vi "Global Controls.vi"() -> ()   [LabVIEW 2020]
uses:
  _controls/PCIe SLM params.ctl
  _controls/PCIe SLM Spots.ctl
  _controls/Spot Params.ctl
  _controls/Exp Params.ctl
  _controls/Global Ctrl Refs.ctl
  _controls/Trapping Laser Control.ctl
  _controls/xiCam.ctl
  <vilib>/userDefined/High Color/IMAQdx.ctl
  _controls/SLM Real World to IMAQ Display Transform.ctl
panel:
  in  "SLM to IMAQ":T1={"Translation"={"X"=255.9856, "Y"=245.976}, "Scalling"={"xScale"=2.61758691206544, "yScale"=-2.61759}}
  in  "Camera Controls":T2={"Exposure Time (ms)"=27, "cam0 Session"="", "Camera ROI"={"Width"=0, "Height"=0, "Offset X"=0, "Offset Y"=0}, "Command"=""} {"Camera ROI"."Offset Y" max=2046 step=2; "Camera ROI"."Offset X" max=2044 step=4; "Camera ROI"."Height" min=2 max=2048 step=2; "Camera ROI"."Width" min=4 max=2048 step=4; "Exposure Time (ms)" min=27 max=500 step=1 scale=27.0..500.0}
  in  "Ventus Controls":T4 caption="Trapping Laser" {"Ventus Power" min=0.0 max=100.0 step=0.1 scale=0.0..100.0}
  in  "Global Ctrl Refs":T5
  in  "Exp Params":T6={"Experiment Type"="Time Series", "Experiment Name"="Experiment_1", "ExpPath"=path "D:/Data", "Save As"="Time Series", "TSFrames"=1000, "TSfps"=1000.0, "Streaming"=FALSE, "tdms ref"=refnum, "frame #"=0, "Full Path"=path "", "PeakOnQueue"=FALSE} {"TSFrames" min=1 step=1; "TSfps" min=0.001 max=90.0 step=0.001 format="%_4g"}
  out "holo_combine":u8[](array[numeric])
  in  "Spots":T7={"Spot Params"=[{"Intensity"=1.0, "Vortex"=0.0, "Phase"=0.0, "X"=0.0, "Y"=0.0, "Z"=0.0}], "Add Spot"=FALSE, "Remove Spot"=FALSE, "Clear All Spots"=FALSE, "Save Spots"=FALSE, "Generate Spots"=FALSE, "Generate Spot Pattern"=""} {"Spot Params"."Z" format="%_4g"; "Spot Params"."Y" format="%_4g"; "Spot Params"."X" format="%_4g"; "Spot Params"."Phase" format="%_4g"; "Spot Params"."Intensity" format="%_4g"}
  out "SLM Params":T9={"Width"=0.0, "Height"=0.0, "Board ID"=0, "Centre Y"=0.46199999999999997, "Centre X"=0.3859999999999999} {"Centre X" format="%.3g"; "Centre Y" format="%.3g"}
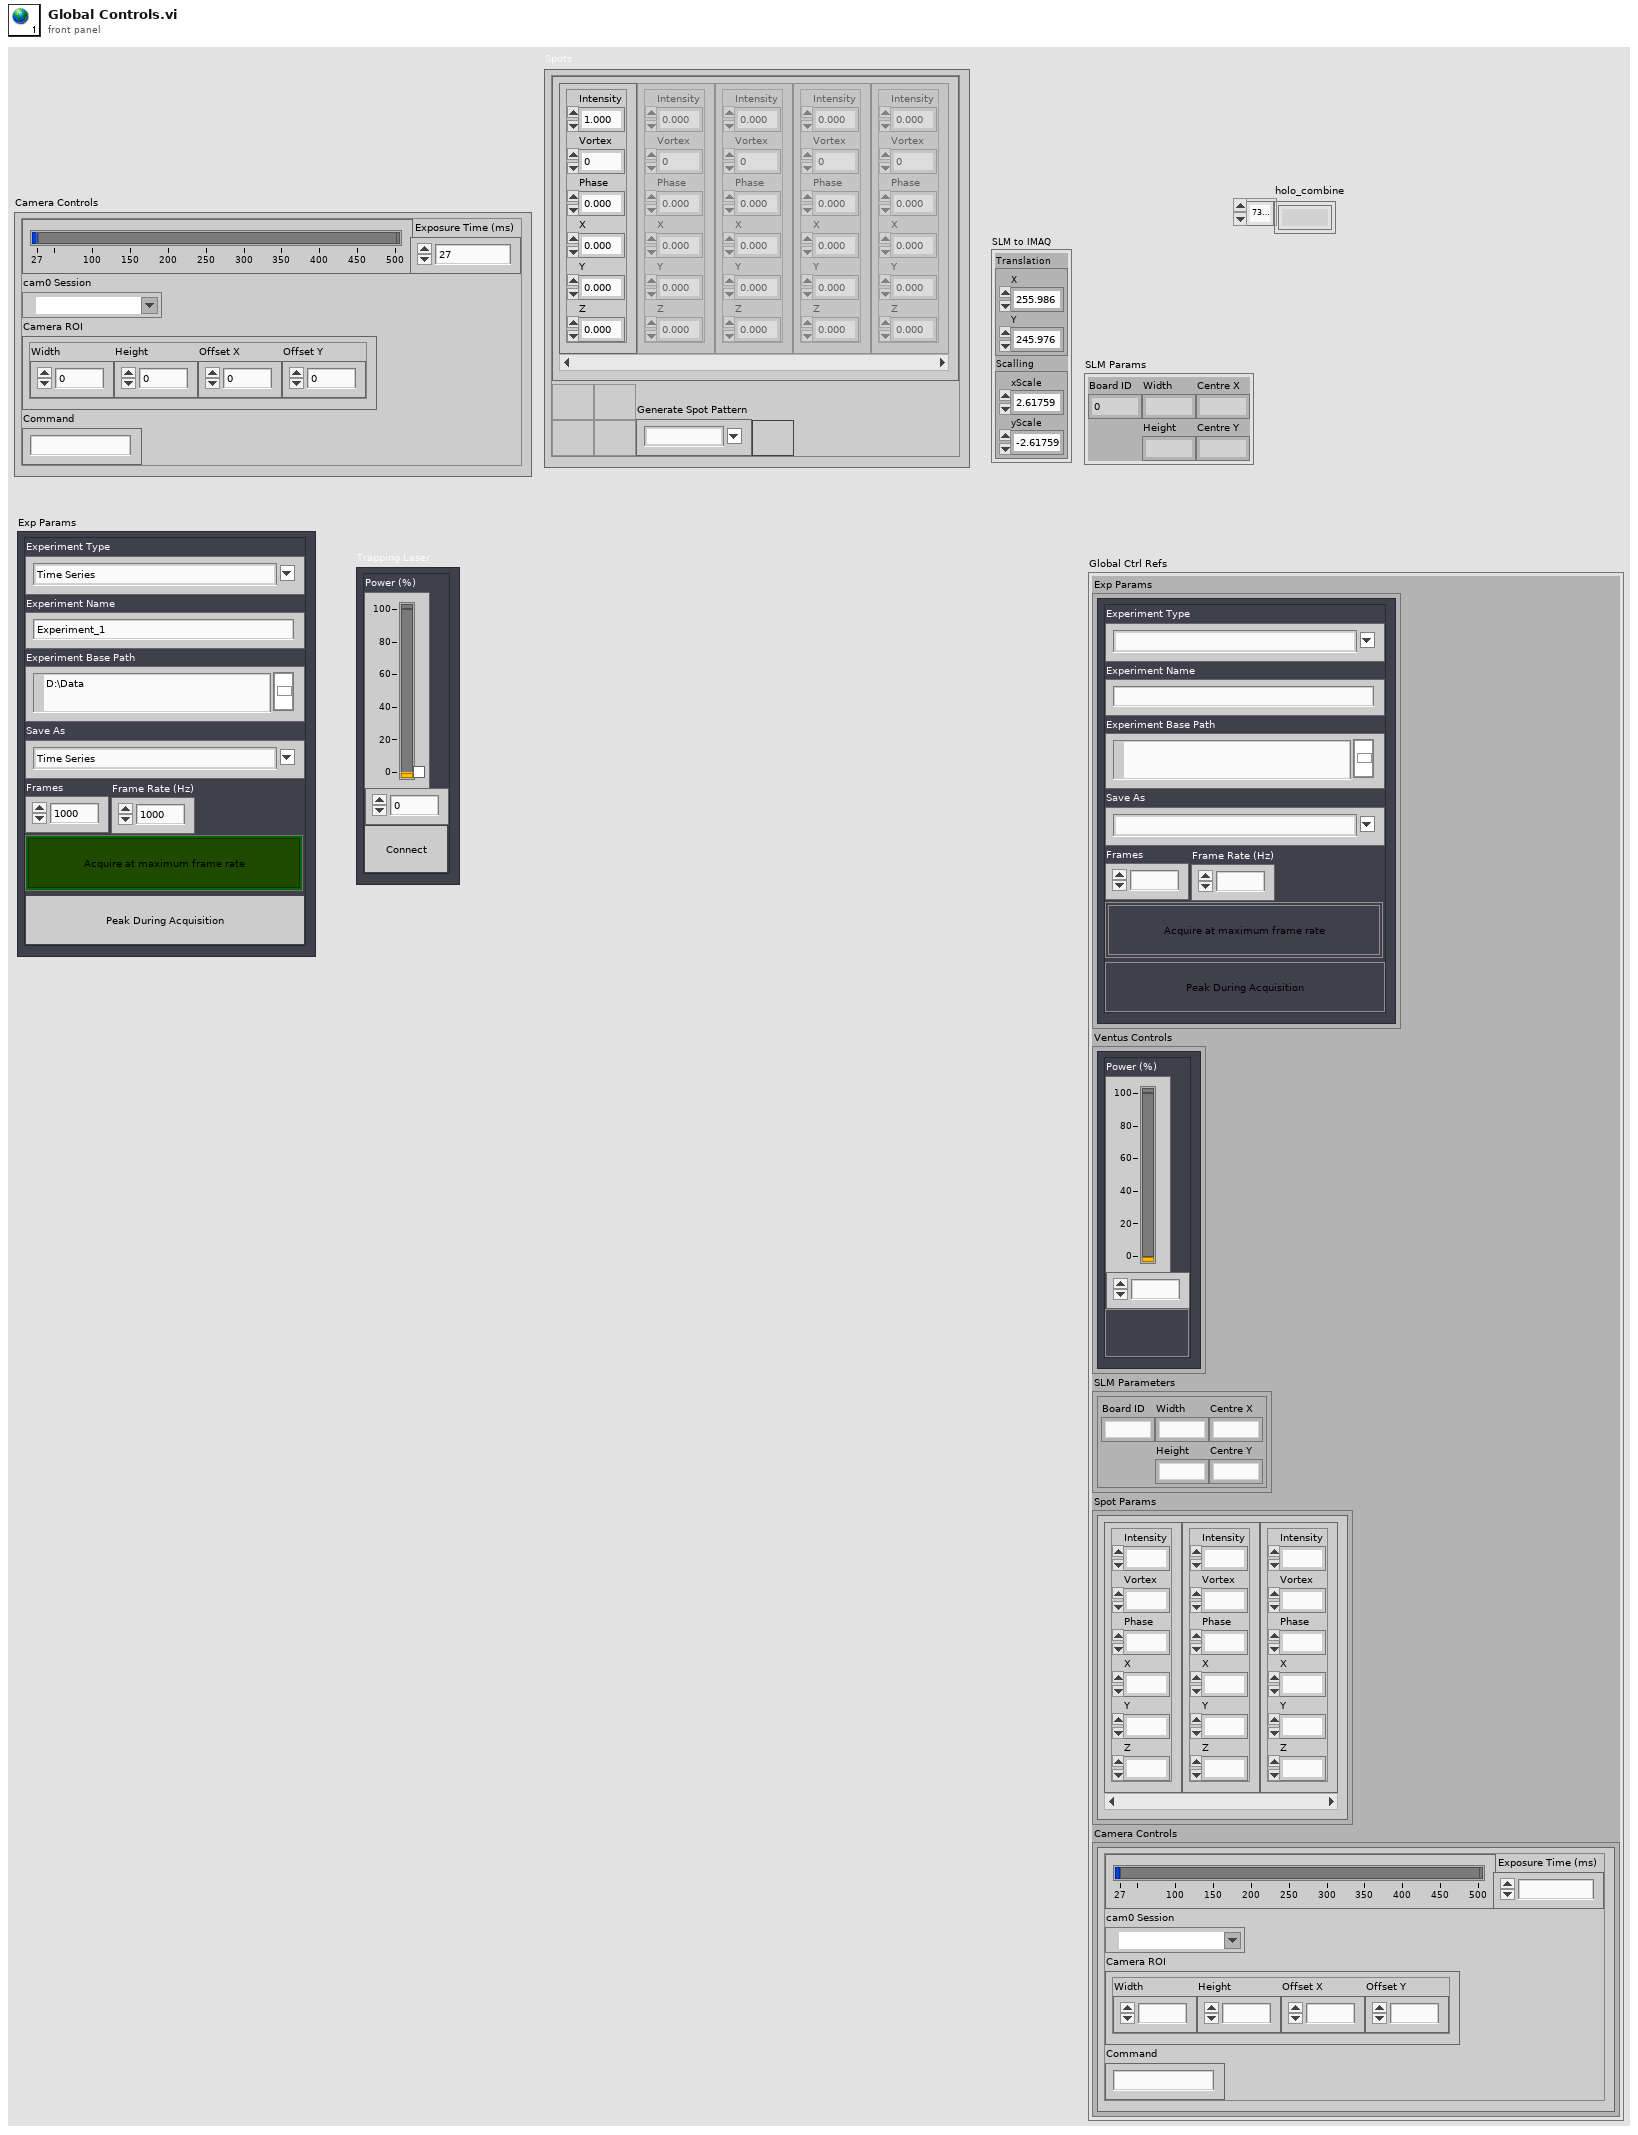
[diagram p1: front panel]
types:
  T1 = typedef "SLM Real World to IMAQ Display Transform.ctl" = cluster{"Translation":cluster{"X":dbl, "Y":dbl}, "Scalling":cluster{"xScale":dbl, "yScale":dbl}}
  T2 = typedef "xiCam.ctl" = cluster{"Exposure Time (ms)":u32, "cam0 Session":T3, "Camera ROI":cluster{"Width":u32, "Height":u32, "Offset X":u32, "Offset Y":u32}, "Command":string}
  T3 = typedef "IMAQdx.ctl" = refnum<k21>
  T4 = typedef "Trapping Laser Control.ctl" = cluster{"Ventus Power":dbl, "Open Serial":bool, "VISA Refnum":refnum<visa-resource-name>}
  T5 = typedef "Global Ctrl Refs.ctl" = cluster{"Exp Params":refnum<vi>, "Ventus Controls":refnum<vi>, "SLM Parameters":refnum<vi>, "Spot Params":refnum<vi>, "Camera Controls":refnum<vi>}
  T6 = typedef "Exp Params.ctl" = cluster{"Experiment Type":string, "Experiment Name":string, "ExpPath":path, "Save As":string, "TSFrames":i32, "TSfps":dbl, "Streaming":bool, "tdms ref":refnum<k34>, "frame #":i64, "Full Path":path, "PeakOnQueue":bool}
  T7 = typedef "PCIe SLM Spots.ctl" = cluster{"Spot Params":T8, "Add Spot":bool, "Remove Spot":bool, "Clear All Spots":bool, "Save Spots":bool, "Generate Spots":bool, "Generate Spot Pattern":string}
  T8 = typedef "Spot Params.ctl" = cluster{"Intensity":dbl, "Vortex":dbl, "Phase":dbl, "X":dbl, "Y":dbl, "Z":dbl}[]
  T9 = typedef "PCIe SLM params.ctl" = cluster{"Width":dbl, "Height":dbl, "Board ID":i32, "Centre Y":dbl, "Centre X":dbl}
diagram:
